vi "Bitshifter.vi"(10 "Bits":u16, 11 "Type":i32) -> (3 "Output":bool)   [LabVIEW 2016]
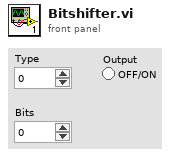
[diagram p1: front panel]
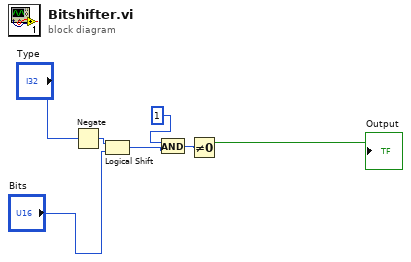
[diagram p0: block diagram]
diagram:
  n1 = Negate(x="Type") -> (-x=w2:i32)
  n2 = Logical Shift(y=w2, x="Bits") -> (x << y=w3:u16)
  n3 = And(x=1, y=w3) -> (x .and. y?=w6:i32)
  n4 = Not Equal To 0?(x=w6) -> (x != 0?=→"Output":bool)
